vi "Init.vi"(8 "Error In":errorcluster, 10 "IConfigure":refnum<class "IConfigure.lvclass">, 11 "object in":refnum<class "Rigol DS1054.lvclass">) -> (0 "Error Out":errorcluster, 3 "object out":refnum<class "Rigol DS1054.lvclass">)   [LabVIEW 2023, in "RIGOL DS1054.lvlib" / "Rigol DS1054.lvclass"]
uses:
  Rigol DS1054.lvclass
  Rigol DS1054.lvclass/Rigol DS1054.ctl
  Hardware_class/Instrument.lvclass
  E:/git/HAL/Scope VISA/Scope VISA.lvclass
  E:/git/HAL/Scope Base/Scope Base.lvclass
  E:/git/HAL/Hardware_class/Instrument.lvclass
  E:/git/HAL/Interfaces/IScope/IScope.lvclass
  E:/git/HAL/Devices/Rigol DS1054/Rigol DS1054.lvclass
  Scope VISA/Scope VISA.lvclass
  Interfaces/IConfigure/IConfigure.lvclass
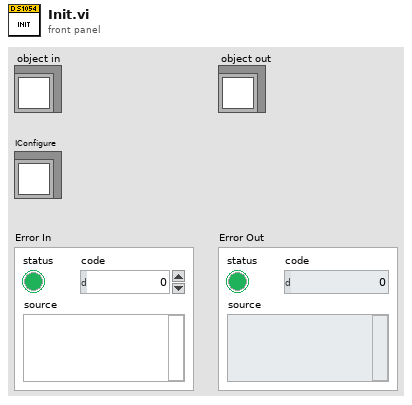
[diagram p1: front panel]
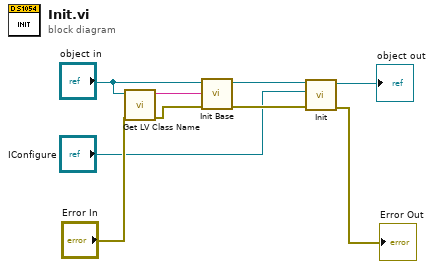
[diagram p0: block diagram]
diagram:
  n1 = call <vilib>:"Get LV Class Name.vi"("error in (no error)"="Error In", "object"="object in") -> ("error out"=w8:errorcluster, "class name"=w9:string)  [unwired: 8 in]
  n2 = call "Init Base.vi"("Error In"=w8, "Device Name"=w9, "object in"="object in") -> ("Error Out"=w6:errorcluster, "object out"=w5:refnum<class "Rigol DS1054.lvclass">)  [unwired: 7 in]
  n3 = call-parent "Init.vi"("Error In"=w6, "HAL.lvlib:IConfigure"="IConfigure", "object in"=w5) -> ("Error Out"=→"Error Out":errorcluster, "object out"=→"object out":refnum<class "Rigol DS1054.lvclass">)  [unwired: 7 in]
